vi "SRListToTable.vi"(7 "Fields to include":T6[](array[typedef]), 8 "Error In":errorcluster, 11 "SR List In":T1[](array[typedef])) -> (0 "Error Out":errorcluster, 3 "2D String Array for Table":string[][](array[string]))   [LabVIEW 2017, in "Client.lvlib" / "UI_API.lvlib"]
uses:
  UI_API.lvlib
  ParserSorter/TypeDefs/AEGroup.ctl
  ParserSorter/TypeDefs/SRLevel.ctl
  ParserSorter/TypeDefs/SRStatus.ctl
  ParserSorter/TypeDefs/SRType.ctl
  ParserSorter/TypeDefs/SRFields.ctl
  ParserSorter/TypeDefs/SRData.ctl
  ParserSorter/ParserSorter.lvlib
panel:
  in  "SR Type":T5
  in  "SR Status":T3
  in  "Prio":T4
  in  "AE Group":T2
  # "Enums for String Conversion Input"
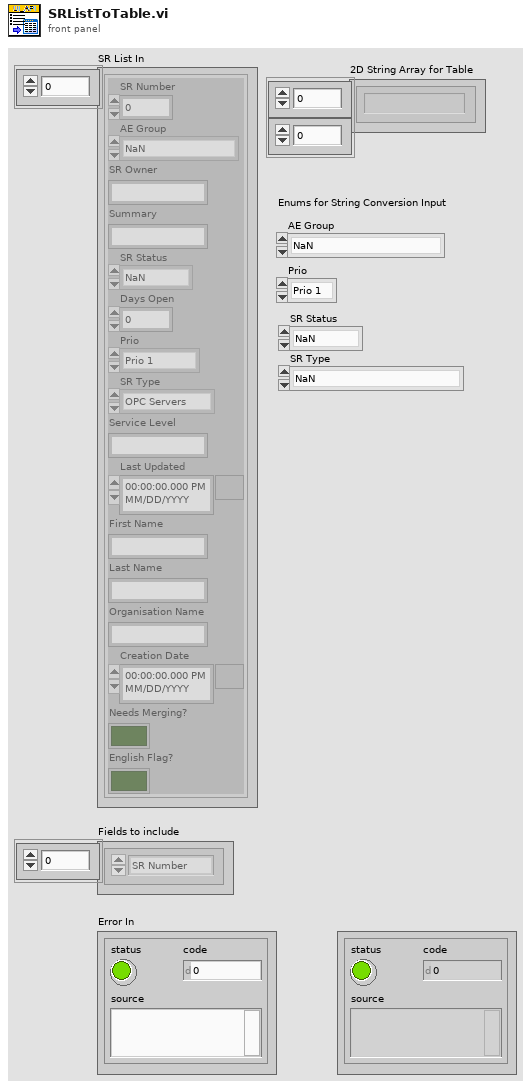
[diagram p1: front panel]
types:
  T1 = typedef "Client.lvlib/ParserSorter.lvlib/SRData.ctl" = cluster{"SR Number":i64, "AE Group":T2, "SR Owner":string, "Summary":string, "SR Status":T3, "Days Open":dbl, "Prio":T4, "SR Type":T5, "Service Level":string, "Last Updated":timestamp, "First Name":string, "Last Name":string, "Organisation Name":string, "Creation Date":timestamp, "Needs Merging?":bool, "English Flag?":bool}
  T2 = typedef "Client.lvlib/ParserSorter.lvlib/AEGroup.ctl" = enum32{"NaN", "AE-Germany", "AE-Poland", "AE-Switzerland", "AE-Czech Republic", "AE-Hungary", "AE-Romania", "AE-Slovakia", "AE-Slovenia"}
  T3 = typedef "Client.lvlib/ParserSorter.lvlib/SRStatus.ctl" = enum32{"NaN", "Caller Abandoned", "Created in Error", "Declined to Purchase Support", "Expired", "Forum Resolved AE", "Forum Resolved Customer", "IN WORK", "IN WORK Collab with AES", "IN WORK Collab with PSE", "IN WORK Collab with SE", "IN WORK Escalation", "IN WORK Customer Added Note", "Open", "Potentially Resolved", "POC Resolved", "Resolved", "RMA Waiting on Customer", "RMA Open", "RMA In Progress", "RMA Closed - DOA", "RMA Closed", "RMA Approved for Return", "Project Complete", "Presumed Resolved", "IN WORK Wait on Customer"}
  T4 = typedef "Client.lvlib/ParserSorter.lvlib/SRLevel.ctl" = enum16{"Prio 1", "Prio 2", "Prio 3", "Prio 4"}
  T5 = typedef "Client.lvlib/ParserSorter.lvlib/SRType.ctl" = enum32{"NaN", "ATE Core Configurations (BYOATE)", "Activation", "BioBench", "CAN", "CM C Series", "Calibration", "Consulting Services", "CounterTimer", "DAQExpress", "DASYLab", "DIAdem", "DMM", "DSA HW", "Digital_IO", "FIRST (NIC Only)", "FieldBus", "FieldPoint", "Functional Savety", "GATI", "GPIB", "HMI and Industrial PCs", "HiQ", "HighSpeedDigital_IO", "IMAQ", "IOTech Vibration", "Industrial Communications", "InsightCM", "LV", "LV CD&Sim", "LV Comms", "LV Controls Add-Ons", "LV Embedded", "LV MathScript RT", "LV NXG", "LV NXT", "LVDSC", "LVFPGA", "LVPDA and LV Touch Panel", "LVRT", "LabWindows_CVI", "Lookout", "MATRIXx", "MStudioDotNet", "MStudioVisualBasic", "MStudioVisualC", "Measure (Legacy)", "Motion", "MultifunctionDAQ", "Multimedia Test HW/SW", "Multisim (EWB)", "NI Update Service", "OPC Servers", "Optical (OSI)", "PXI Controllers, Chassis, MXI", "PXI Timing and Sync", "Power Supplies and SMUs", "Powertrain Controls", "RAID", "RF", "RF Software", "RIO", "SC Express", "SCC", "SCXI", "SPEEDY-33 (Hyperception)", "STS", "ScopeDigitizers", "Serial", "Signal Sources", "SignalCondOther", "SignalExpress", "Software Defined Intruments", "Sound and Vibration SW", "Switch Executive", "Switches", "TestStand", "USRP", "Ultiboard (EWB)", "VBench", "VI Logger", "VXI_MXI", "VeriStand", "VisionSW", "VolumeLicenseMgr", "WSN", "Web UI Builder", "myRIO"}
  T6 = typedef "Client.lvlib/ParserSorter.lvlib/SRFields.ctl" = enum16{"SR Number", "AE Group", "SR Owner", "Summary", "SR Status", "Days Open", "Prio", "SR Type", "Service Level", "Last Updated", "First Name", "Last Name", "Organisation Name", "Creation Date", "Needs Merging?", "English Flag?"}
  T7 = cluster{"Strings []":string[], "Strings []":string[], "Strings []":string[], "Strings []":string[]}
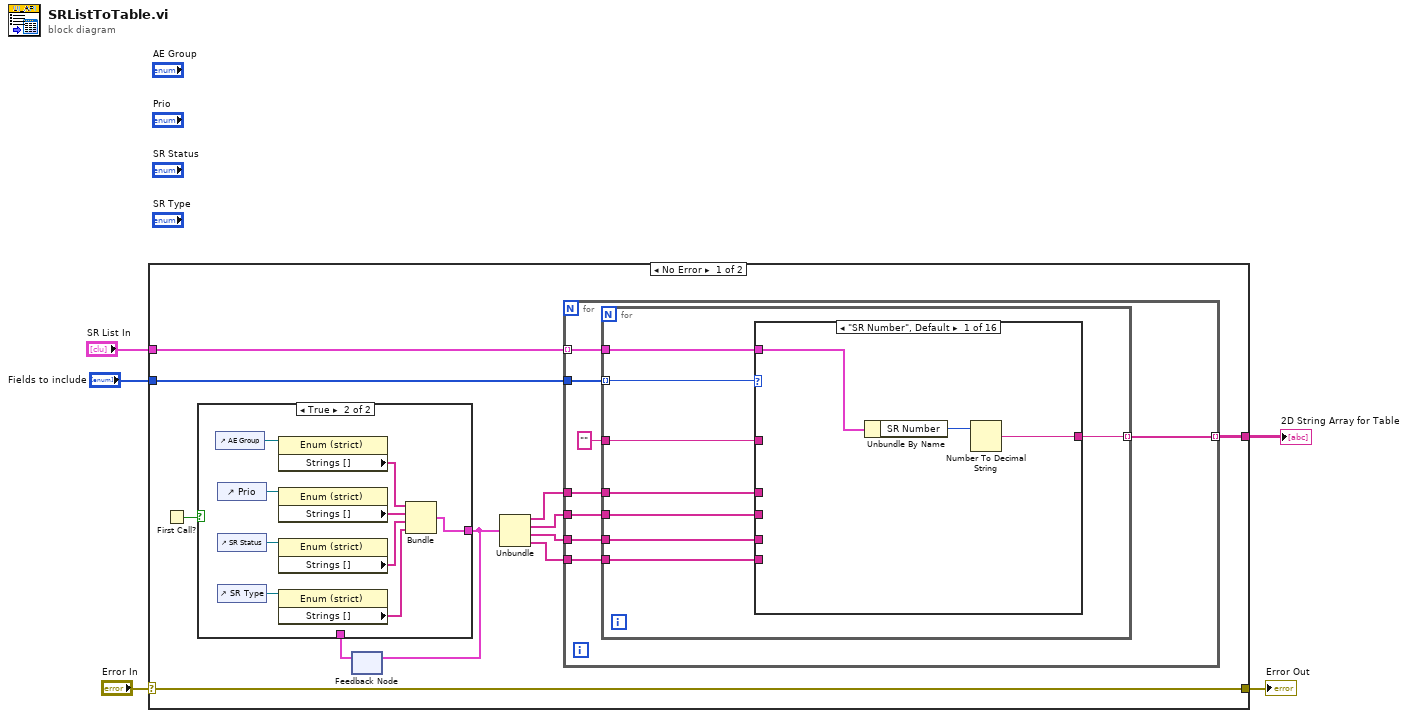
[diagram p0: block diagram]
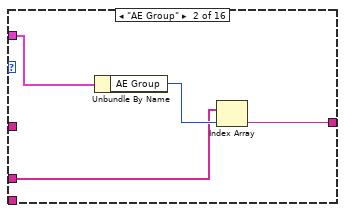
[diagram p2: hidden frame]
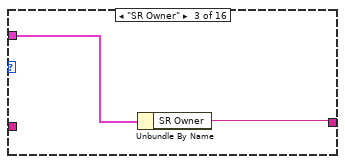
[diagram p3: hidden frame]
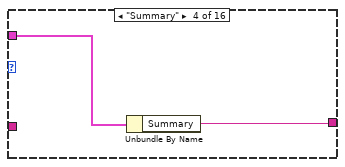
[diagram p4: hidden frame]
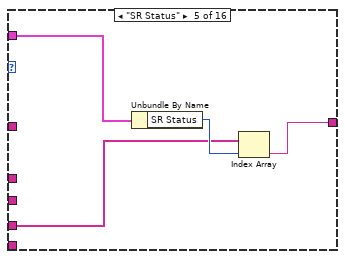
[diagram p5: hidden frame]
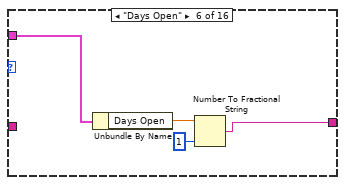
[diagram p6: hidden frame]
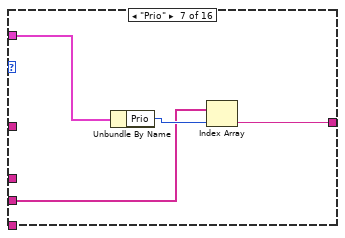
[diagram p7: hidden frame]
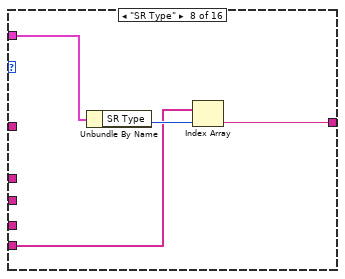
[diagram p8: hidden frame]
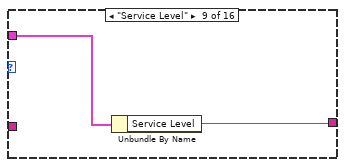
[diagram p9: hidden frame]
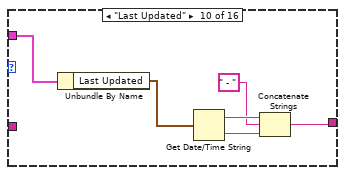
[diagram p10: hidden frame]
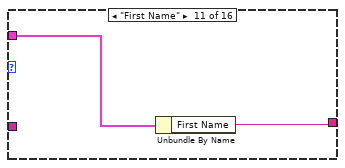
[diagram p11: hidden frame]
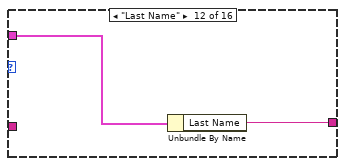
[diagram p12: hidden frame]
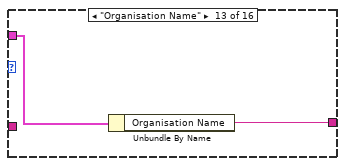
[diagram p13: hidden frame]
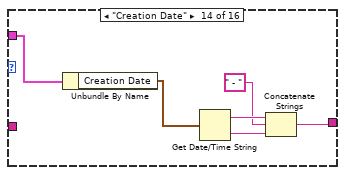
[diagram p14: hidden frame]
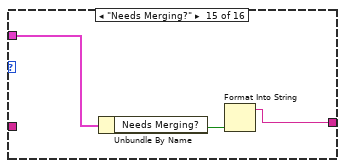
[diagram p15: hidden frame]
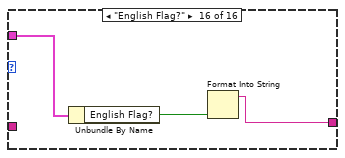
[diagram p16: hidden frame]
diagram:
  n1 = case shown="No Error" "Error In" {
    selector: "Error In" -> [w14 w96]
    tunnel: "SR List In" -> [w16 _]
    tunnel: "Fields to include" -> [w15 _]
    tunnel: [w14 w96] -> w3
    tunnel: [w13 _] -> w2
    frame No Error {
      n2 = First Call?() -> (First Call?: T/F=w10:bool)
      n3 = feedback #1() -> (w11:T7)  [unwired: 1 in]
      n4 = case shown="True" w10 {
        tunnel: [w86 w87] -> w12
        tunnel: w11 -> [w86 _]
        frame False {
        }
        frame True {
          n5 = control-ref of="AE Group"() -> (w92:refnum<vi>)
          n6 = control-ref of="Prio"() -> (w93:refnum<vi>)
          n7 = control-ref of="SR Status"() -> (w94:refnum<vi>)
          n8 = control-ref of="SR Type"() -> (w95:refnum<vi>)
          n9 = property class="Enum (strict)"(reference=w92) -> ("Strings []"=w91:string[])  [unwired: 1 in, 2 out]
          n10 = property class="Enum (strict)"(reference=w93) -> ("Strings []"=w90:string[])  [unwired: 1 in, 2 out]
          n11 = property class="Enum (strict)"(reference=w94) -> ("Strings []"=w89:string[])  [unwired: 1 in, 2 out]
          n12 = property class="Enum (strict)"(reference=w95) -> ("Strings []"=w88:string[])  [unwired: 1 in, 2 out]
          n13 = Bundle("Strings []"=w91, "Strings []"=w90, "Strings []"=w89, "Strings []"=w88) -> (w87:T7)  [unwired: 1 in]
        }
      }
      n14 = feedback-in #1(w12) -> ()
      n15 = Unbundle(w12) -> ("Strings []"=w9:string[], "Strings []"=w8:string[], "Strings []"=w7:string[], "Strings []"=w6:string[])
      n16 = for {
        tunnel: w16 -> [w23] mode=indexing
        tunnel: w15 -> [w24]
        tunnel: w9 -> [w21]
        tunnel: w8 -> [w20]
        tunnel: w7 -> [w19]
        tunnel: w6 -> [w18]
        tunnel: [w17] -> w13 mode=indexing
        n17 = for {
          tunnel: w24 -> [w32] mode=indexing
          tunnel: w23 -> [w31]
          tunnel: "" -> [w30]
          tunnel: w21 -> [w29]
          tunnel: w20 -> [w28]
          tunnel: w19 -> [w27]
          tunnel: w18 -> [w26]
          tunnel: [w25] -> w17 mode=indexing
          n18 = case shown="\"SR Number\", Default" w32 {
            tunnel: w31 -> [w35 w39 w41 w43 w47 w51 w55 w58 w61 w67 w69 w71 w73 w75 w82 w85]
            tunnel: w30 -> [_ _ _ _ _ _ _ _ _ _ _ _ _ _ _ _]
            tunnel: w29 -> [_ w37 _ _ _ _ _ _ _ _ _ _ _ _ _ _]
            tunnel: w28 -> [_ _ _ _ _ _ w53 _ _ _ _ _ _ _ _ _]
            tunnel: w27 -> [_ _ _ _ w45 _ _ _ _ _ _ _ _ _ _ _]
            tunnel: w26 -> [_ _ _ _ _ _ _ w57 _ _ _ _ _ _ _ _]
            tunnel: [w33 w36 w40 w42 w44 w49 w52 w56 w60 w62 w68 w70 w72 w74 w80 w83] -> w25
            frame "SR Number", Default {
              n19 = Unbundle By Name(w35) -> ("SR Number"=w34:i64)
              n20 = Number To Decimal String(number=w34) -> (decimal integer string=w33:string)  [unwired: 1 in]
            }
            frame "AE Group" {
              n21 = Unbundle By Name(w39) -> ("AE Group"=w38:T2)
              n22 = Index Array(array=w37, index=w38) -> (element=w36:string)
            }
            frame "SR Owner" {
              n23 = Unbundle By Name(w41) -> ("SR Owner"=w40:string)
            }
            frame "Summary" {
              n24 = Unbundle By Name(w43) -> ("Summary"=w42:string)
            }
            frame "SR Status" {
              n25 = Unbundle By Name(w47) -> ("SR Status"=w46:T3)
              n26 = Index Array(array=w45, index=w46) -> (element=w44:string)
            }
            frame "Days Open" {
              n27 = Unbundle By Name(w51) -> ("Days Open"=w50:dbl)
              n28 = Number To Fractional String(number=w50, precision (6)=i16 1) -> (F-format string=w49:string)  [unwired: 2 in]
            }
            frame "Prio" {
              n29 = Unbundle By Name(w55) -> ("Prio"=w54:T4)
              n30 = Index Array(array=w53, index=w54) -> (element=w52:string)
            }
            frame "SR Type" {
              n31 = Unbundle By Name(w58) -> ("SR Type"=w59:T5)
              n32 = Index Array(array=w57, index=w59) -> (element=w56:string)
            }
            frame "Service Level" {
              n33 = Unbundle By Name(w61) -> ("Service Level"=w60:string)
            }
            frame "Last Updated" {
              n34 = Unbundle By Name(w67) -> ("Last Updated"=w66:timestamp)
              n35 = Get Date/Time String(seconds (now)=w66) -> (date string=w65:string, time string=w64:string)  [unwired: 2 in]
              n36 = Concatenate Strings(w65, " - ", w64) -> (w62:string)
            }
            frame "First Name" {
              n37 = Unbundle By Name(w69) -> ("First Name"=w68:string)
            }
            frame "Last Name" {
              n38 = Unbundle By Name(w71) -> ("Last Name"=w70:string)
            }
            frame "Organisation Name" {
              n39 = Unbundle By Name(w73) -> ("Organisation Name"=w72:string)
            }
            frame "Creation Date" {
              n40 = Unbundle By Name(w75) -> ("Creation Date"=w79:timestamp)
              n41 = Get Date/Time String(seconds (now)=w79) -> (date string=w78:string, time string=w77:string)  [unwired: 2 in]
              n42 = Concatenate Strings(w78, " - ", w77) -> (w74:string)
            }
            frame "Needs Merging?" {
              n43 = Unbundle By Name(w82) -> ("Needs Merging?"=w81:bool)
              n44 = Format Into String(w81) -> (resulting string=w80:string)  [unwired: 3 in, 1 out]
            }
            frame "English Flag?" {
              n45 = Unbundle By Name(w85) -> ("English Flag?"=w84:bool)
              n46 = Format Into String(w84) -> (resulting string=w83:string)  [unwired: 3 in, 1 out]
            }
          }
        }
      }
    }
    frame Error {
    }
  }
  "2D String Array for Table" <- w2
  "Error Out" <- w3
